vi "PHIXdll.vi"(8 "error in (no error)":errorcluster, 11 "Inputs":T1) -> (0 "error out":errorcluster, 3 "phixx":dbl)   [LabVIEW 2016]
doc: "subroutine PHIXdll(itau, idel, tau, del, z, phixx)\n\nCompute reduced Helmholtz energy or a derivative as functions of dimensionless temperature and density by\ncalling the appropriate mixture model.\n\nThe Helmholtz energy consists of ideal-gas and residual (real- gas) terms. The residual term consists of idealsolution\nand mixing terms. This routine calculates only the residual term.\n\nINPUTS:\nitau -- Flag specifying order of temperature derivative to calculate\nidel -- Flag specifying order of density derivative to calculate When itau = 0 and idel = 0, compute A/RT. When itau \n = 0 and idel = 1, compute 1st density derivative. When itau= 1 and idel = 1, compute cross derivative. etc.\ntau -- Dimensionless temperature (Tr/T)\ndel -- Dimensionless density (D/Dr)\nz -- Composition (array of mole fractions)\n\nOUTPUTS:\nphixx -- Residual (real-gas) part of the Helmholtz energy, or one\n of its derivatives (as specified by itau and idel),\n in reduced form (A/RT), multiplied by tau**itau*delta**idelta"
uses:
  REFPROP.DLL
panel:
  # "REFPROP-PHIXdll.vi"
  # "void  PHIXdll(int32_t *itau, int32_t *idel, double *tau, double *del, double *z, double *phixx)"
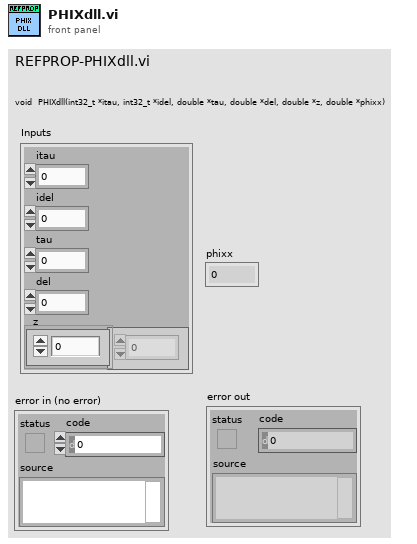
[diagram p1: front panel]
types:
  T1 = cluster{"itau":i32, "idel":i32, "tau":dbl, "del":dbl, "z":dbl[]}
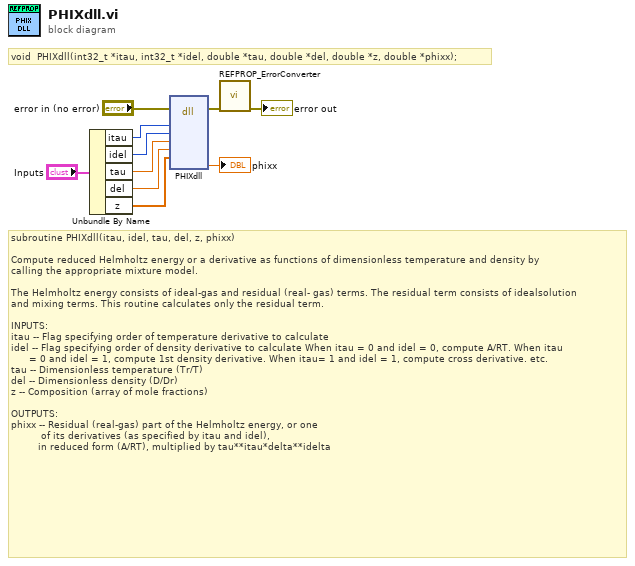
[diagram p0: block diagram]
diagram:
  # "void  PHIXdll(int32_t *itau, int32_t *idel, double *tau, double *del, double *z, double *phixx);"
  # "subroutine PHIXdll(itau, idel, tau, del, z, phixx)\n\nCompute reduced Helmholtz energy or a derivative as functions of dimensionless temperature and density by\ncalling the appropriate mixture model.\n\nThe Helmholtz energy consists of ideal-gas and residual (real- gas) terms. The residual term consists of idealsolution\nand mixing terms. This routine calculates only the residual term.\n\nINPUTS:\nitau -- Flag specifying order of temperature derivative to calculate\nidel -- Flag specifying order of density derivative to calculate When itau = 0 and idel = 0, compute A/RT. When itau   \n      = 0 and idel = 1, compute 1st density derivative. When itau= 1 and idel = 1, compute cross derivative. etc.\ntau -- Dimensionless temperature (Tr/T)\ndel -- Dimensionless density (D/Dr)\nz -- Composition (array of mole fractions)\n\nOUTPUTS:\nphixx -- Residual (real-gas) part of the Helmholtz energy, or one\n          of its derivatives (as specified by itau and idel),\n         in reduced form (A/RT), multiplied by tau**itau*delta**idelta"
  n1 = Unbundle By Name("Inputs") -> ("itau"=w5:i32, "idel"=w4:i32, "tau"=w3:dbl, "del"=w2:dbl, "z"=w1:dbl[])
  n2 = dll-call lib="S:/009 - Testing/02 - Performance Testing/REFPROP/REFPROP.*" fn="PHIXdll"(error in="error in (no error)", "itau"=w5, "idel"=w4, "tau"=w3, "del"=w2, "z"=w1) -> (error out=w9:errorcluster, "phixx"=→"phixx":dbl)  [unwired: 9 in, 1 out]
  n3 = call "REFPROP_ErrorConverter.vi"("error in (no error)"=w9) -> ("error out"=→"error out":errorcluster)  [unwired: 10 in]
